vi "Thermal_Camera_IMGTempExtract.vi"(0 "img dst":T1, 5 "img process dst":T1, 7 "Image in":T1, 9 "Mouse pos":cluster{"X":i32, "Y":i32}, 11 "error in (no error)":errorcluster) -> (3 "appended array":i8[][](array[numeric]), 4 "img out":T1, 6 "temp":sgl, 8 "temp str":string, 10 "Mouse pos dup":cluster{"X":i32, "Y":i32}, 15 "error out":errorcluster)   [LabVIEW 2020]
uses:
  <vilib>/vision/Image Controls.llb/IMAQ Image.ctl
  <vilib>/vision/NI_Vision_Development_Module.lvlib
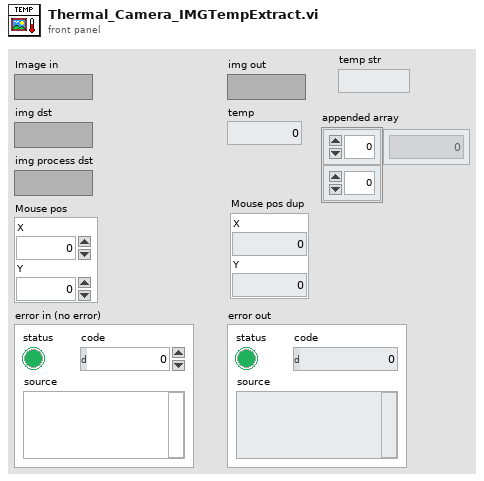
[diagram p1: front panel]
types:
  T1 = typedef "IMAQ Image.ctl" = refnum<image>
  T2 = cluster{"histogram":u32[], "Minimal Value":sgl, "Maximal Value":sgl, "Starting Value":sgl, "Interval Width":sgl, "Mean Value":sgl, "Standard  Variation":sgl, "Area (pixels)":i32}
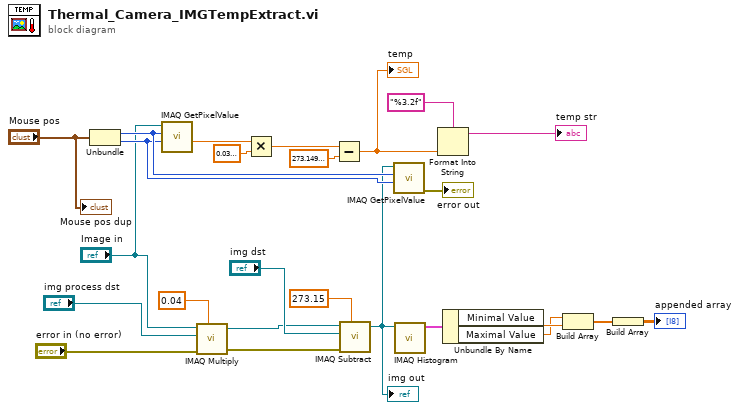
[diagram p0: block diagram]
diagram:
  n1 = Unbundle("Mouse pos") -> ("X"=w14:i32, "Y"=w13:i32)
  n2 = call "IMAQ GetPixelValue"("Image"="Image in", "X Coordinate"=w14, "Y Coordinate"=w13) -> ("Pixel Value (Float)"=w12:sgl)  [unwired: 3 in, 4 out]
  n3 = call "IMAQ Multiply"("Image Src A"="Image in", "Constant"=0.04, "Image Dst"="img process dst", "error in (no error)"="error in (no error)") -> ("Image Dst Out"=w18:T1, "error out"=w23:errorcluster)  [unwired: 3 in]
  n4 = Multiply(x=w12, y=sgl 0.04) -> (x*y=w10:sgl)
  n5 = Subtract(x=w10, y=sgl 273.15) -> (x-y=w7:sgl)
  "temp" <- w7
  n6 = call "IMAQ Subtract"("Image Src A"=w18, "Constant"=273.15, "Image Dst"="img dst", "error in (no error)"=w23) -> ("Image Dst Out"=w6:T1)  [unwired: 3 in, 1 out]
  "img out" <- w6
  n7 = call "IMAQ GetPixelValue"("Image"=w6, "X Coordinate"=w14, "Y Coordinate"=w13) -> ("error out"=→"error out":errorcluster)  [unwired: 3 in, 4 out]
  n8 = call "IMAQ Histogram"("Image"=w6) -> ("Histogram Report"=w5:T2)  [unwired: 9 in, 1 out]
  n9 = Format Into String(format string="%3.2f", w7) -> (resulting string=→"temp str":string)  [unwired: 2 in, 1 out]
  n10 = Unbundle By Name(w5) -> ("Minimal Value"=w4:sgl, "Maximal Value"=w2:sgl)
  n11 = Build Array(w2, w4) -> (w3:sgl[])
  n12 = Build Array(w3) -> (→"appended array":sgl[][])
  "Mouse pos dup" <- "Mouse pos"
